vi "CaLabPut_Main.vi"(0 "PV Names":string[](array[string]), 1 "Data Type":i32(ring) items=["String", "SGL", "DBL", "I8", "I16", "I32", "I64"], 2 "variable PV names (F)":bool, 3 "Timeout (3)":dbl=3.0, 5 "Values [String]":string[][](array[string]), 7 "Values [DBL]":dbl[][](array[numeric]), 9 "Values [I64]":i64[][](array[numeric]), 11 "Error in (no error)":errorcluster, 12 "Synchronous":bool) -> (4 "PV Names (dup)":string[](array[string]), 6 "Status":bool, 10 "PV Errors":errorcluster[](array[cluster]), 15 "Error out":errorcluster)   [LabVIEW 2018]
doc: "This is a polymorphic VI for setting values of EPICS variables.\n\nINPUT:\n <b>PV name(s)</b>\n name of EPICS variable\n <b>value(s)</b>\n Boolean value OR Double value OR Double array OR String array\n <b>timeout</b>\n optional\n timeout for Channel Access requests\n <b>error in</b>\n <b>buffer size (since version 1.3 without function)</b>\n <b>synchronous</b>\n optional\n TRUE=synchronous; FALSE=asynchronous\n synchronous = writes value(s) after waiting for end of record processing\n <b>ValueSetsInColumns</b>\n optional\n TRUE = use columns for value sets instead of rows\n\nOUTPUT:\n <b>PV name(s)</b>\n name of EPICS variable\n </b>status</b>\n FALSE: request successful\n TRUE: warnings or errors\n <b>errors</b>\n resulting errors of all put commands\n <b>error out</b>\n global io error"
uses:
  <userlib>/caLab/lib/caLab.dll
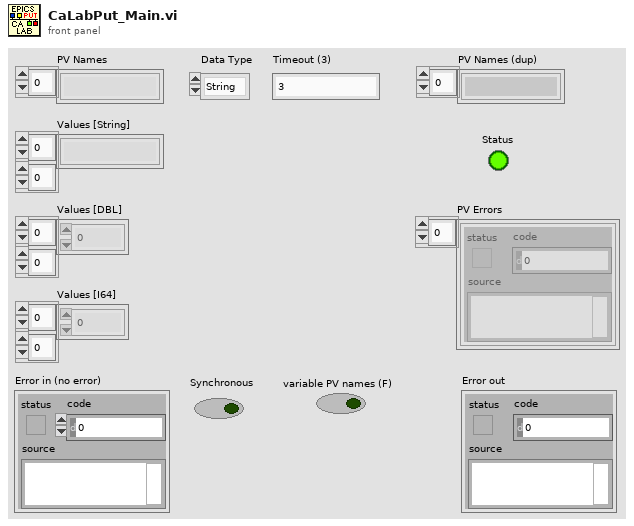
[diagram p1: front panel]
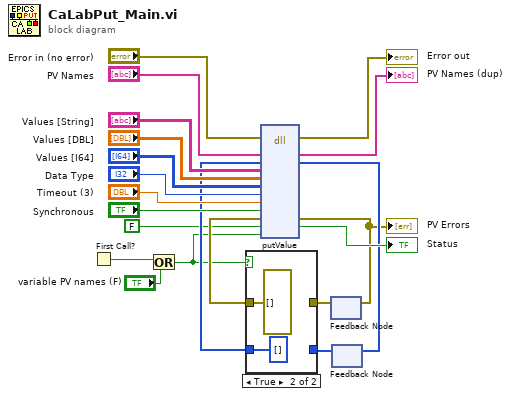
[diagram p0: block diagram]
diagram:
  n1 = First Call?() -> (First Call?: T/F=w2:bool)
  n2 = Or(x=w2, y="variable PV names (F)") -> (x .or. y?=w1:bool)
  n3 = feedback #1() -> (w9:errorcluster[])  [unwired: 1 out]
  n4 = feedback #2() -> (w7:u64[])  [unwired: 1 out]
  n5 = case shown="True" w1 {
    tunnel: [w23 errorcluster[] []] -> w10
    tunnel: w9 -> [w23 _]
    tunnel: [w22 u64[] [] ("IndexArray")] -> w8
    tunnel: w7 -> [w22 _]
    frame False {
    }
    frame True {
    }
  }
  n6 = dll-call lib="D:/Program Files (x86)/National Instruments/LabVIEW 2018/user.lib/caLab/lib/calab.dll" fn="putValue" ("caLabPut")(error in="Error in (no error)", "PVNameArray"="PV Names", "IndexArray"=w8, "ValueArrayString"="Values [String]", "ValueArrayDoubleFloat"="Values [DBL]", "ValueArrayI64"="Values [I64]", "DataType"="Data Type", "Timeout"="Timeout (3)", "Synchronous"="Synchronous", "ErrorArray"=w10, "Status"=FALSE, "FirstCall"=w1) -> (error out=→"Error out":errorcluster, "PVNameArray"=→"PV Names (dup)":string[], "IndexArray"=w6:u64[], "ErrorArray"=w5:errorcluster[], "Status"=→"Status":bool)  [unwired: 8 in, 3 out]
  "PV Errors" <- w5
  n7 = feedback-in #1(w5) -> ()
  n8 = feedback-in #2(w6) -> ()
